vi "Moving STFT PtByPt.vi"() -> ()   [LabVIEW 2023]
doc: "This VI performs real-time Joint-Time Frequency Analysis (JTFA) using the STFT Spectrogram PtByPt VI. The signal is simulated by a sine wave plus Gaussian noise."
uses:
  <vilib>/ptbypt/NI_PtbyPt.lvlib
panel:
  in  "window selector":i32(ring) items=["Hanning", "Hamming", "Blackman", "Exact Blackman", "Blackman-Harris"]
  out "Waveform Chart":dbl(graph)=-0.6173802395237638
  in  "noise level":dbl(slide)=0.1 scale=0.0..1.0 scale format="%#.2f"
  in  "frequency":dbl(slide)=0.1 scale=0.0..0.5 scale format="%#.2f"
  out "Moving STFT":dbl[][](graph)
  in  "sample length":i32=200
  in  "window length":i32=100 format="%0.0f"
  in  "Stop":bool
  # "Overview: Performs real-time Joint-Time Frequency Analysis (JTFA) using the STFT Spectrogram PtByPt VI.\nRequirement: LabVIEW Full Development System\nInstructions:\n1. Run the VI.\n2. Change the frequency and noise level of the signal and observe the results in the Moving STFT intensity graph.\n3. Change the window length, sample length, and window selector to change the behavior of the STFT Spectrogram PtByPt VI.\n4. Click Stop to stop the VI."
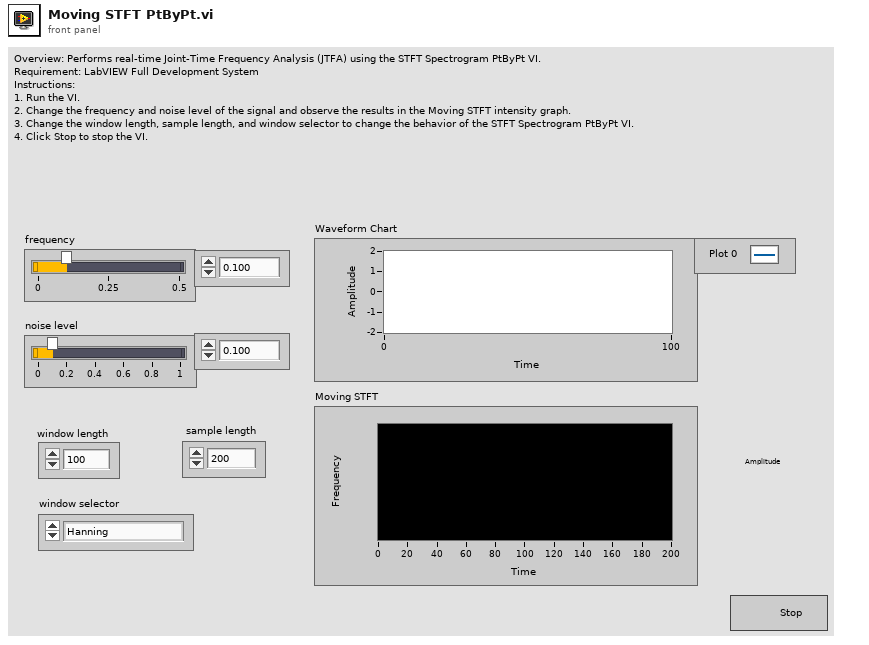
[diagram p1: front panel]
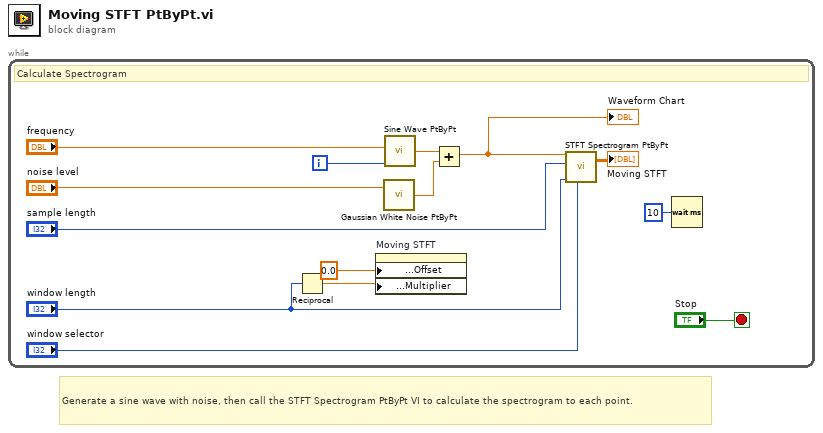
[diagram p0: block diagram]
diagram:
  # "Generate a sine wave with noise, then call the STFT Spectrogram PtByPt VI to calculate the spectrogram to each point."
  n1 = while {
    i -> [w1]
    stop <- "Stop" stop-if-true
    # "Calculate Spectrogram"
    n2 = Reciprocal(x="window length") -> (1/x=w3:dbl)
    n3 = property on="Moving STFT" class="IntGraph (strict)"("Y Scale.Offset and Multiplier:Offset"=0.0, "Y Scale.Offset and Multiplier:Multiplier"=w3) -> ()  [unwired: 2 in, 2 out]
    n4 = call <vilib>:"Gaussian White Noise PtByPt.vi"("standard deviation"="noise level") -> ("Gaussian white noise"=w11:dbl)  [unwired: 2 in]
    n5 = call <vilib>:"Sine Wave PtByPt.vi"("time"=w1, "frequency"="frequency") -> ("sine wave"=w12:dbl)  [unwired: 2 in]
    n6 = Add(x=w12, y=w11) -> (x+y=w7:dbl)
    "Waveform Chart" <- w7
    n7 = call <vilib>:"STFT Spectrogram PtByPt.vi"("window selector"="window selector", "window length"="window length", "sample length"="sample length", "x"=w7) -> ("STFT Spectrogram {X}"=→"Moving STFT":dbl[][])  [unwired: 2 in, 1 out]
    n8 = Wait (ms)(milliseconds to wait=u32 10) -> ()  [unwired: 1 out]
  }
